vi "PixyCam_Loop.vi"(4 "error in":errorcluster, 6 "stop":bool, 7 "PixyCamDevRef":T1) -> (0 "error out":errorcluster, 3 "PixyCamDevRef Out":T1)   [LabVIEW 2016, in "PixyCam_LabVIEW.lvlib"]
uses:
  PixyCam_LabVIEW.lvlib
  Private/PixyCam_DevRef.ctl
  Private/PixyCam_SPI_DevRef.ctl
  <vilib>/Rock Robotics/WPI/SPI/WPI_SPIDevRef.ctl
  <vilib>/Rock Robotics/SystemInterfaces/spilib/spi_bus.ctl
  Private/PixyCam_CommMode.ctl
  Private/PixyCam_TargetData.ctl
  <vilib>/Utility/SystemLogging/NI_SystemLogging.lvlib
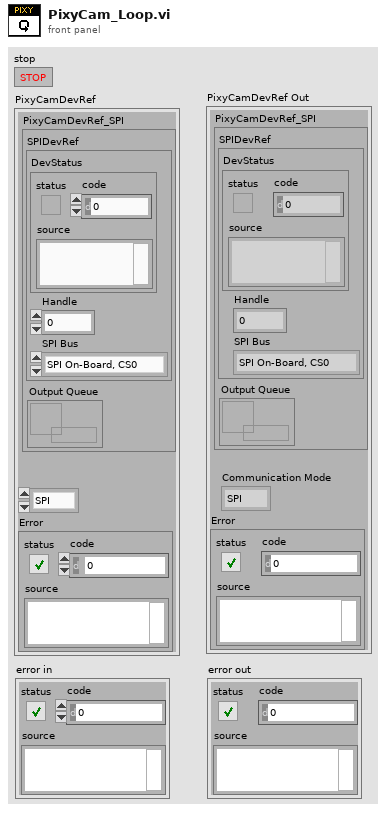
[diagram p1: front panel]
types:
  T1 = typedef "PixyCam_LabVIEW.lvlib/PixyCam_DevRef.ctl" = cluster{"PixyCamDevRef_SPI":T2, "Communication Mode":T5, "Error":errorcluster}
  T2 = typedef "PixyCam_LabVIEW.lvlib/PixyCam_SPI_DevRef.ctl" = cluster{"SPIDevRef":T3, "Output Queue":refnum<queue>}
  T3 = typedef "WPI_SPIDevRef.ctl" = cluster{"DevStatus":errorcluster, "Handle":i32, "SPI Bus":T4}
  T4 = typedef "spi_bus.ctl" = enum16{"SPI On-Board, CS0", "SPI On-Board, CS1", "SPI On-Board, CS2", "SPI On-Board, CS3", "SPI MXP", "Invalid"}
  T5 = typedef "PixyCam_LabVIEW.lvlib/PixyCam_CommMode.ctl" = enum16{"SPI", "I2C", "UART", "Analog", "Digital"}
  T6 = typedef "PixyCam_LabVIEW.lvlib/PixyCam_TargetData.ctl" = cluster{"Target Type":u16, "Checksum":u16, "Signature Number":u16, "X Center":u16, "Y Center":u16, "Width":u16, "Height":u16, "Angle":u16}
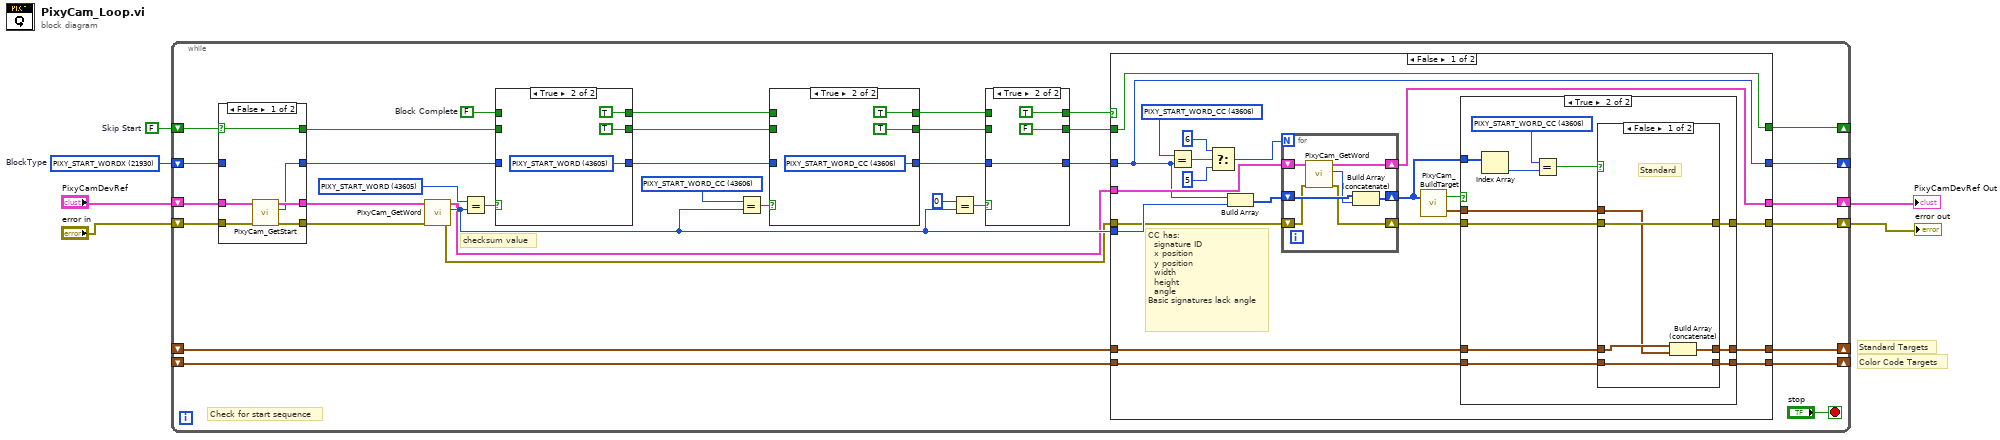
[diagram p0: block diagram]
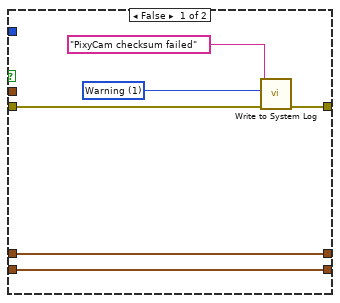
[diagram p2: hidden frame]
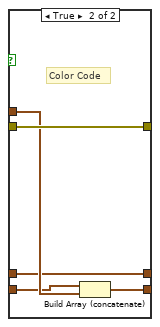
[diagram p3: hidden frame]
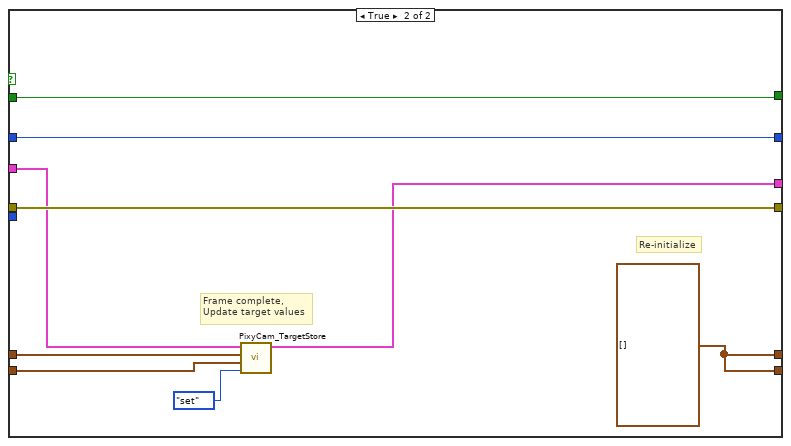
[diagram p4: hidden frame]
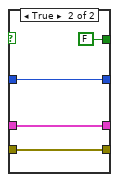
[diagram p8: hidden frame]
diagram:
  w1 = u16 21930 items=["PIXY_START_WORD"=43605, "PIXY_START_WORD_CC"=43606, "PIXY_START_WORDX"=21930]  # BlockType
  w2 = FALSE  # Skip Start
  # "Color Code Targets"
  # "Standard Targets"
  n1 = while {
    shift-right: [w7] -> w3
    shift-left: "PixyCamDevRef" -> [w41]
    shift-right: [w14] -> w4
    shift-left: "error in" -> [w40]
    shift-right: [w10] -> _
    shift-left: w1 -> [w35]
    shift-right: [w8] -> _
    shift-left: w2 -> [w37]
    shift-right: [w15] -> _
    shift-left: _ -> [w11]
    shift-right: [w13] -> _
    shift-left: _ -> [w12]
    stop <- "stop" stop-if-true
    w26 = FALSE  # Block Complete
    w28 = u16 43606 items=["PIXY_START_WORD"=43605, "PIXY_START_WORD_CC"=43606, "PIXY_START_WORDX"=21930] ("IDWord")
    w36 = u16 43605 items=["PIXY_START_WORD"=43605, "PIXY_START_WORD_CC"=43606, "PIXY_START_WORDX"=21930] ("IDWord")
    # "checksum value"
    # "Check for start sequence"
    n2 = case shown="False" w37 {
      selector: w37 -> [w125 _]
      tunnel: w41 -> [w130 w134]
      tunnel: w40 -> [w129 w133]
      tunnel: [w128 w134] -> w38
      tunnel: [w127 w133] -> w39
      tunnel: w35 -> [_ w132]
      tunnel: [w126 w132] -> w33
      tunnel: [w125 FALSE] -> w32
      frame False {
        n3 = call "PixyCam_GetStart.vi"("error in"=w129, "PixyCamDevRef"=w130) -> ("error out"=w127:errorcluster, "WordType"=w126:u16, "PixyCamDevRef Out"=w128:T1)  [unwired: 3 in]
      }
      frame True {
      }
    }
    n4 = call "PixyCam_GetWord.vi"("error in"=w39, "PixyCamDevRef"=w38) -> ("error out"=w16:errorcluster, "Word Out"=w19:u16, "PixyCamDevRefOut"=w17:T1)  [unwired: 3 in]
    n5 = Equal?(x=w36, y=w19) -> (x = y?=w34:bool)
    n6 = case shown="True" w34 {
      tunnel: w33 -> [w121 _]
      tunnel: [w121 w123] -> w30
      tunnel: [w120 TRUE] -> w31
      tunnel: w32 -> [w120 _]
      tunnel: [w119 TRUE] -> w27
      tunnel: w26 -> [w119 _]
      frame False {
      }
      frame True {
        w123 = u16 43605 items=["PIXY_START_WORD"=43605, "PIXY_START_WORD_CC"=43606, "PIXY_START_WORDX"=21930] ("IDWord")
      }
    }
    n7 = Equal?(x=w28, y=w19) -> (x = y?=w29:bool)
    n8 = case shown="True" w29 {
      tunnel: w30 -> [w115 _]
      tunnel: [w115 w117] -> w23
      tunnel: [w114 TRUE] -> w24
      tunnel: w31 -> [w114 _]
      tunnel: w27 -> [w113 _]
      tunnel: [w113 TRUE ("Block Complete")] -> w25
      frame False {
      }
      frame True {
        w117 = u16 43606 items=["PIXY_START_WORD"=43605, "PIXY_START_WORD_CC"=43606, "PIXY_START_WORDX"=21930] ("IDWord")
      }
    }
    n9 = Equal?(x=u16 0, y=w19) -> (x = y?=w22:bool)
    n10 = case shown="True" w22 {
      tunnel: w23 -> [w109 w110]
      tunnel: [w109 w110] -> w18
      tunnel: [w108 FALSE] -> w9
      tunnel: w24 -> [w108 _]
      tunnel: w25 -> [w107 _]
      tunnel: [w107 TRUE ("Block Complete")] -> w20
      frame False {
      }
      frame True {
      }
    }
    n11 = case shown="False" w20 {
      tunnel: w19 -> [w56 _]
      tunnel: w18 -> [w44 w100]
      tunnel: w17 -> [w57 w104]
      tunnel: w16 -> [w55 w106]
      tunnel: [w51 w105] -> w15
      tunnel: [w50 w106] -> w14
      tunnel: [w48 w105] -> w13
      tunnel: w12 -> [w47 w103]
      tunnel: w11 -> [w46 w102]
      tunnel: [w44 w100] -> w10
      tunnel: [w45 w99] -> w8
      tunnel: w9 -> [w45 w99]
      tunnel: [w43 w98] -> w7
      frame False {
        w63 = u16 43606 items=["PIXY_START_WORD"=43605, "PIXY_START_WORD_CC"=43606, "PIXY_START_WORDX"=21930] ("IDWord")
        # "CC has:\n  signature ID\n  x position\n  y position\n  width\n  height\n  angle\nBasic signatures lack angle"
        n12 = Equal?(x=w63, y=w44) -> (x = y?=w62:bool)
        n13 = Select(t=6, s=w62, f=5) -> (s? t:f=w59:i32)
        n14 = Build Array(w44, w56) -> (w58:u16[])
        n15 = for {
          N: w59 -> [_]
          shift-right: [w94] -> w49
          shift-left: w58 -> [w96]
          shift-right: [w93] -> w53
          shift-left: w55 -> [w92]
          shift-right: [w91] -> w43
          shift-left: w57 -> [w97]
          n16 = call "PixyCam_GetWord.vi"("error in"=w92, "PixyCamDevRef"=w97) -> ("error out"=w93:errorcluster, "Word Out"=w95:u16, "PixyCamDevRefOut"=w91:T1)  [unwired: 3 in]
          n17 = Build Array (concatenate)(w96, w95) -> (w94:u16[])
        }
        n18 = call "PixyCam_BuildTarget.vi"("RawData"=w49) -> ("Target"=w52:T6, "Valid Checksum"=w54:bool)  [unwired: 1 in]
        n19 = case shown="True" w54 {
          tunnel: w53 -> [w69 w80]
          tunnel: w52 -> [_ w74]
          tunnel: [w64 w73] -> w51
          tunnel: [w66 w79] -> w50
          tunnel: w49 -> [_ w78]
          tunnel: [w65 w72] -> w48
          tunnel: w47 -> [w65 w71]
          tunnel: w46 -> [w64 w70]
          frame False {
            w68 = 1 items=["Error", "Warning", "Informational"] ("severity")
            n20 = call <vilib>:"Write to System Log.vi"("error in (no error)"=w69, "severity"=w68, "message"="PixyCam checksum failed") -> ("error out"=w66:errorcluster)  [unwired: 8 in]
          }
          frame True {
            w76 = u16 43606 items=["PIXY_START_WORD"=43605, "PIXY_START_WORD_CC"=43606, "PIXY_START_WORDX"=21930] ("IDWord")
            n21 = Index Array(array=w78) -> (element=w77:u16)  [unwired: 1 in]
            n22 = Equal?(x=w76, y=w77) -> (x = y?=w75:bool)
            n23 = case shown="False" w75 {
              tunnel: w80 -> [w85 w90]
              tunnel: [w85 w90] -> w79
              tunnel: w74 -> [w82 w89]
              tunnel: [w81 w87] -> w73
              tunnel: [w83 w86] -> w72
              tunnel: w71 -> [w84 w86]
              tunnel: w70 -> [w81 w88]
              frame False {
                # "Standard"
                n24 = Build Array (concatenate)(w84, w82) -> (w83:T6[])
              }
              frame True {
                # "Color Code"
                n25 = Build Array (concatenate)(w88, w89) -> (w87:T6[])
              }
            }
          }
        }
      }
      frame True {
        w105 = T6[] []
        # "Frame complete,\nUpdate target values"
        # "Re-initialize"
        n26 = call "PixyCam_TargetStore.vi"("Operation"=enum16{"set", "get"}."set", "ColorCodeTargets Set"=w102, "StandardTargets Set"=w103, "PixyCamDevRef"=w104) -> ("PixyCamDevRef Out"=w98:T1)  [unwired: 1 in, 2 out]
      }
    }
  }
  "error out" <- w4
  "PixyCamDevRef Out" <- w3
